vi "DAQ.vi"   [LabVIEW 2017, in "DAQ.lvlib"]
uses:
  DAQ.lvlib
  DAQ.Data.ctl
  <vilib>/DAQmx/read.llb/DAQmx Read (Analog 2D DBL NChan NSamp).vi
  <vilib>/DAQmx/read.llb/DAQmx Read (Digital 1D Bool NChan 1Samp 1Line).vi
  <vilib>/DAQmx/write.llb/DAQmx Write (Digital 1D Bool NChan 1Samp 1Line).vi
  <vilib>/DAQmx/miscellaneous.llb/DAQmx Fill In Error Info.vi
  DAQ.Global.vi
  Communication/Communication.lvlib
types:
  T1 = typedef "DAQ.lvlib/DAQ.Data.ctl" = cluster{"AI":refnum<k21>, "DI":refnum<k21>, "DO":refnum<k21>, "Save AI":bool}
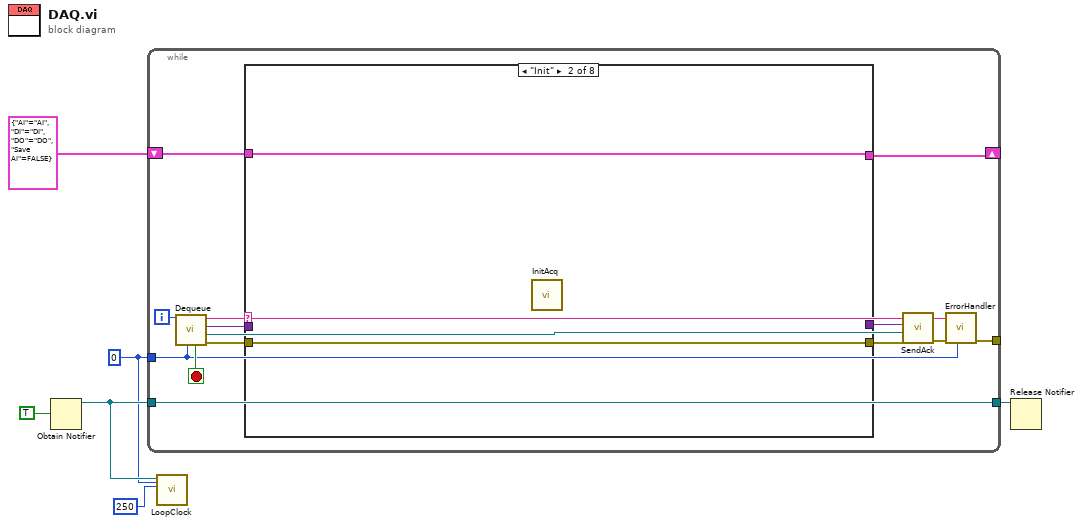
[diagram p0: block diagram]
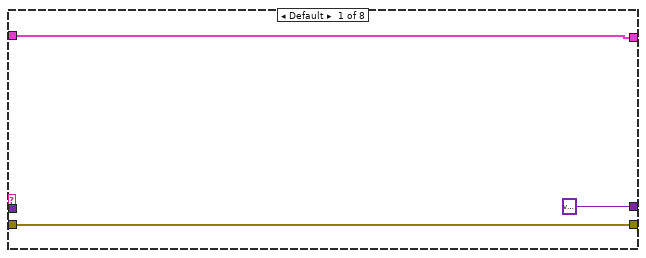
[diagram p2: hidden frame]
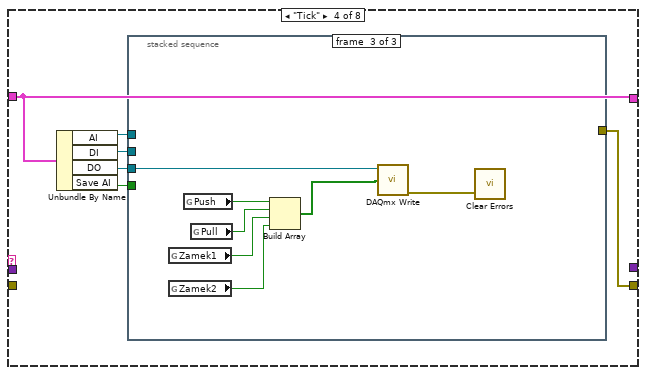
[diagram p4: hidden frame]
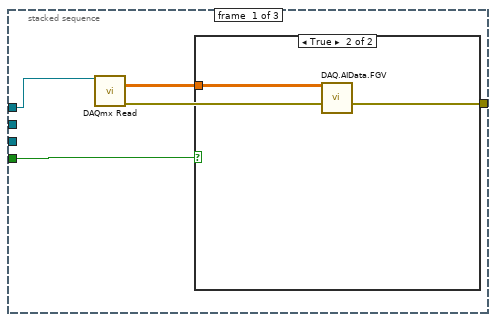
[diagram p5: hidden frame]
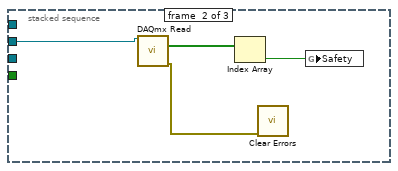
[diagram p7: hidden frame]
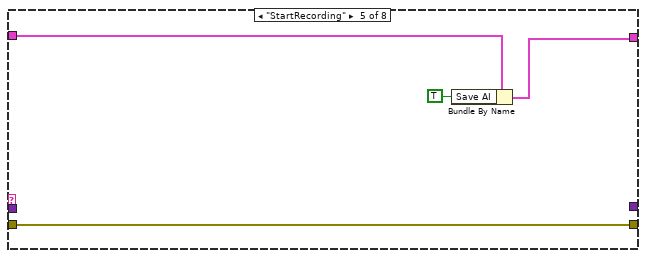
[diagram p8: hidden frame]
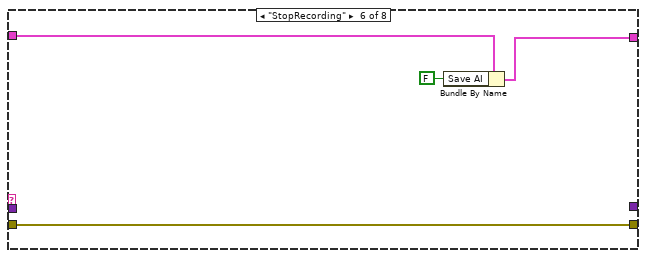
[diagram p9: hidden frame]
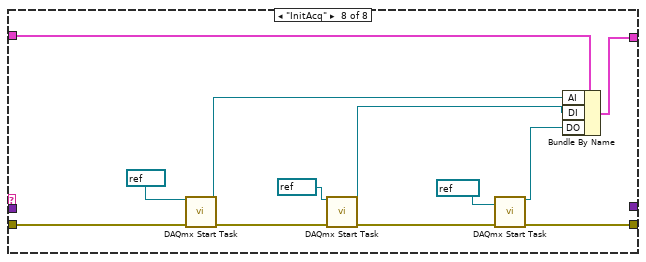
[diagram p11: hidden frame]
diagram:
  w2 = 0
  n1 = Obtain Notifier(notification data type=TRUE) -> (notifier out=w6:refnum<notifier>)  [unwired: 3 in, 2 out]
  n2 = while {
    tunnel: w6 -> [w18]
    tunnel: [w18] -> w4
    tunnel: w2 -> [w11]
    tunnel: [w13] -> _
    shift-right: [w7] -> _
    shift-left: T1 {"AI"="AI", "DI"="DI", "DO"="DO", "Save AI"=FALSE} -> [w8]
    i -> [w12]
    stop <- w20 stop-if-true
    n3 = call "Dequeue.vi"("Instance"=w11, "Loop Counter"=w12) -> ("error out"=w16:errorcluster, "ResponseNotifcation"=w17:refnum<notifier>, "Data"=w19:variant, "Msg"=w10:string, "Exit?"=w20:bool)  [unwired: 5 in]
    n4 = case shown="\"Init\"" w10 {
      tunnel: w19 -> [_ _ _ _ _ _ _ _]
      tunnel: w16 -> [w23 w25 w27 _ w53 w54 w59 w62]
      tunnel: [variant _ _ _ _ _ _ _] -> w15
      tunnel: [w23 w25 w27 w28 w53 w54 w59 w71] -> w9
      tunnel: w8 -> [w21 w24 w26 w29 w52 w57 w58 w70]
      tunnel: [w21 w24 w26 w29 w50 w56 w58 w66] -> w7
      frame Default {
      }
      frame "Init" {
        n5 = call "InitAcq.vi"() -> ()  [unwired: 11 in, 1 out]
      }
      frame "Exit" {
      }
      frame "Tick" {
        n6 = Unbundle By Name(w29) -> ("AI"=w33:refnum<k21>, "DI"=w31:refnum<k21>, "DO"=w30:refnum<k21>, "Save AI"=w32:bool)
        n7 = stacked-sequence {
          tunnel: w33 -> [w36 _ _]
          tunnel: w32 -> [w37 _ _]
          tunnel: w31 -> [_ w42 _]
          tunnel: w30 -> [_ _ w49]
          tunnel: [w34 _ _] -> w28
          frame #0 {
            n8 = call-poly <vilib>:"DAQmx Read.vi"("task/channels in"=w36) -> ("data"=w35:dbl[][], "error out"=w34:errorcluster)  [unwired: 12 in, 1 out]
            n9 = case shown="True" w37 {
              tunnel: w35 -> [_ w38]
              frame False {
              }
              frame True {
                n10 = call "DAQ.AIData.FGV.vi"("Data In"=w38) -> ()  [unwired: 9 in, 2 out]
              }
            }
          }
          frame #1 {
            n11 = call-poly <vilib>:"DAQmx Read.vi"("task/channels in"=w42) -> ("data"=w41:bool[], "error out"=w39:errorcluster)  [unwired: 12 in, 1 out]
            n12 = Index Array(array=w41) -> (element=w40:bool)  [unwired: 1 in]
            n13 = call <vilib>:"Clear Errors.vi"("error in (no error)"=w39) -> ()  [unwired: 5 in, 2 out]
            n14 = global write "DAQ.Global.vi" "Safety"(w40) -> ()
          }
          frame #2 {
            n15 = global read "DAQ.Global.vi" "Zamek1"() -> (w46:bool)
            n16 = global read "DAQ.Global.vi" "Zamek2"() -> (w45:bool)
            n17 = global read "DAQ.Global.vi" "Push"() -> (w48:bool)
            n18 = global read "DAQ.Global.vi" "Pull"() -> (w47:bool)
            n19 = Build Array(w48, w47, w46, w45) -> (w44:bool[])
            n20 = call-poly <vilib>:"DAQmx Write.vi"("task/channels in"=w49, "data"=w44) -> ("error out"=w43:errorcluster)  [unwired: 11 in, 2 out]
            n21 = call <vilib>:"Clear Errors.vi"("error in (no error)"=w43) -> ()  [unwired: 5 in, 2 out]
          }
        }
      }
      frame "StartRecording" {
        n22 = Bundle By Name(cluster=w52, "Save AI"=TRUE) -> (w50:T1)
      }
      frame "StopRecording" {
        n23 = Bundle By Name(cluster=w57, "Save AI"=FALSE) -> (w56:T1)
      }
      frame "Error" {
      }
      frame "InitAcq" {
        n24 = call <vilib>:"DAQmx Start Task.vi"("task/channels in"=refnum<k21> "AI" ("task in"), "error in"=w62) -> ("task out"=w69:refnum<k21>, "error out"=w61:errorcluster)  [unwired: 12 in]
        n25 = call <vilib>:"DAQmx Start Task.vi"("task/channels in"=refnum<k21> "DI" ("task out"), "error in"=w61) -> ("task out"=w68:refnum<k21>, "error out"=w60:errorcluster)  [unwired: 12 in]
        n26 = call <vilib>:"DAQmx Start Task.vi"("task/channels in"=refnum<k21> "DO" ("task out"), "error in"=w60) -> ("task out"=w67:refnum<k21>, "error out"=w71:errorcluster)  [unwired: 12 in]
        n27 = Bundle By Name(cluster=w70, "AI"=w69, "DI"=w68, "DO"=w67) -> (w66:T1)
      }
    }
    n28 = call "SendAck.vi"("error in (no error)"=w9, "Ack"=w17, "Variant"=w15) -> ("error out"=w14:errorcluster)  [unwired: 8 in]
    n29 = call "ErrorHandler.vi"("Instance"=w11, "error in (no error)"=w14, "Msg"=w10) -> ("error out"=w13:errorcluster)  [unwired: 8 in]
  }
  n30 = call "LoopClock.vi"("Instance"=w2, "timeout in ms (-1)"=250, "Notifier in"=w6) -> ()  [unwired: 9 in]
  n31 = Release Notifier(notifier=w4) -> ()  [unwired: 2 in, 3 out]
